vi "Read_Write_Text_File.vi"(0 "File_Path":path, 7 "Data":string, 11 "Error_In":errorcluster, 13 "File_Operation_Select":T1=enum."Close") -> (4 "Data":string, 15 "Error_Out":errorcluster)   [LabVIEW 2021]
doc: "Used to open, read, write and close the File"
uses:
  Controls/File_Operation_Select.ctl
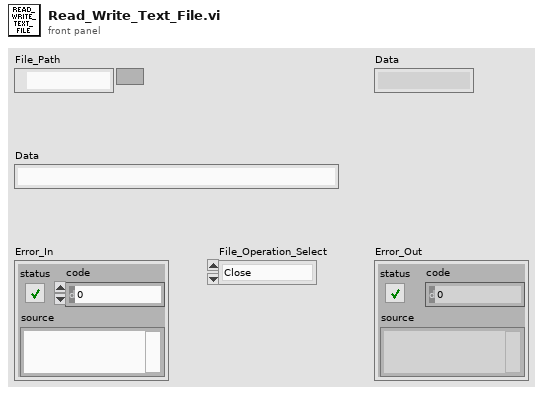
[diagram p1: front panel]
types:
  T1 = typedef "File_Operation_Select.ctl" = enum16{"Open", "Write", "Read", "Close"}
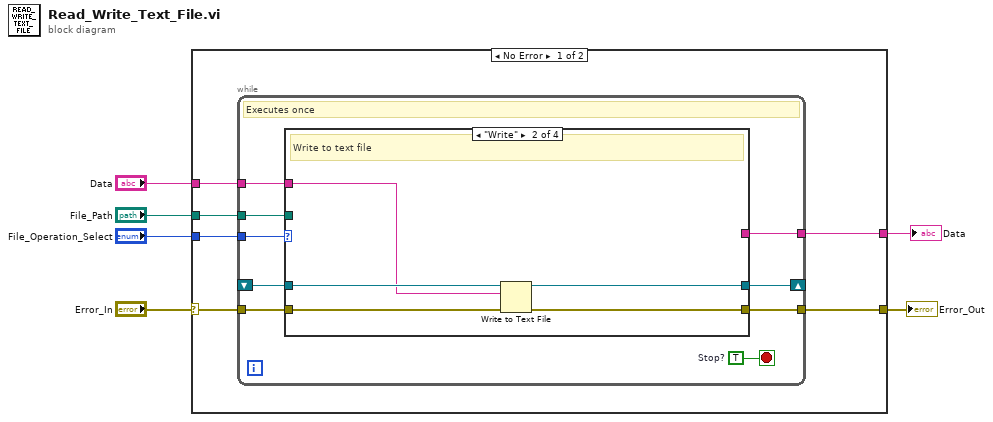
[diagram p0: block diagram]
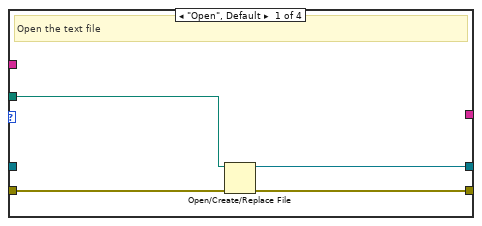
[diagram p2: hidden frame]
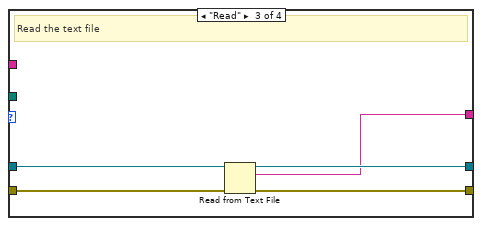
[diagram p3: hidden frame]
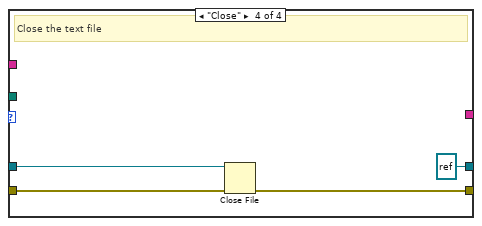
[diagram p4: hidden frame]
diagram:
  n1 = case shown="No Error" "Error_In" {
    selector: "Error_In" -> [w11 w40]
    tunnel: "File_Operation_Select" -> [w12 _]
    tunnel: [w10 w40] -> w4
    tunnel: "File_Path" -> [w9 _]
    tunnel: "Data" -> [w8 _]
    tunnel: [w7 _] -> w1
    frame No Error {
      n2 = while {
        tunnel: w12 -> [w21]
        tunnel: w11 -> [w20]
        tunnel: [w19] -> w10
        tunnel: w9 -> [w18]
        shift-right: [w17] -> _
        shift-left: _ -> [w16]
        tunnel: w8 -> [w15]
        tunnel: [w13] -> w7
        stop <- w14 stop-if-true
        w14 = TRUE  # Stop?
        # "Executes once"
        n3 = case shown="\"Write\"" w21 {
          tunnel: w20 -> [w25 w30 w35 w39]
          tunnel: [w24 w29 w34 w38] -> w19
          tunnel: w18 -> [w23 _ _ _]
          tunnel: [w22 w26 w32 refnum<file> refnum ("refnum out")] -> w17
          tunnel: w16 -> [_ w28 w33 w37]
          tunnel: w15 -> [_ w27 _ _]
          tunnel: [_ _ w31 _] -> w13
          frame "Open", Default {
            # "Open the text file"
            n4 = Open/Create/Replace File(file path (use dialog)=w23, error in=w25) -> (refnum out=w22:refnum<file>, error out=w24:errorcluster)  [unwired: 4 in, 1 out]
          }
          frame "Write" {
            # "Write to text file"
            n5 = Write to Text File(file (use dialog)=w28, text=w27, error in=w30) -> (refnum out=w26:refnum<file>, error out=w29:errorcluster)  [unwired: 1 in, 1 out]
          }
          frame "Read" {
            # "Read the text file"
            n6 = Read from Text File(file (use dialog)=w33, error in=w35) -> (refnum out=w32:refnum<file>, text=w31:string, error out=w34:errorcluster)  [unwired: 2 in, 1 out]
          }
          frame "Close" {
            # "Close the text file"
            n7 = Close File(refnum=w37, error in=w39) -> (error out=w38:errorcluster)  [unwired: 1 out]
          }
        }
      }
    }
    frame Error {
    }
  }
  "Error_Out" <- w4
  "Data" <- w1
